vi "ReadRCMFileToTree.vi"(7 "tree control":refnum<class "TreeControl.lvclass">, 8 "error in (no error)":errorcluster) -> (0 "error out":errorcluster, 3 "rcm file path out":path)   [LabVIEW 2009]
uses:
  Support/Tree Control/Library/TreeControl.lvclass
  Support/MSXML/Public/MSXML Document/msxml document.lvclass
  Support/MSXML/Public/MSXML Node/msxml node.lvclass
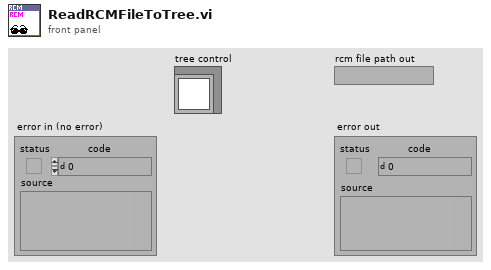
[diagram p1: front panel]
types:
  T1 = typedef "MSXML.lvlib/Attributes__slk_msxml.ctl" = T2[]
  T2 = typedef "MSXML.lvlib/Attribute__slk_msxml.ctl" = cluster{"name":string, "value":string}
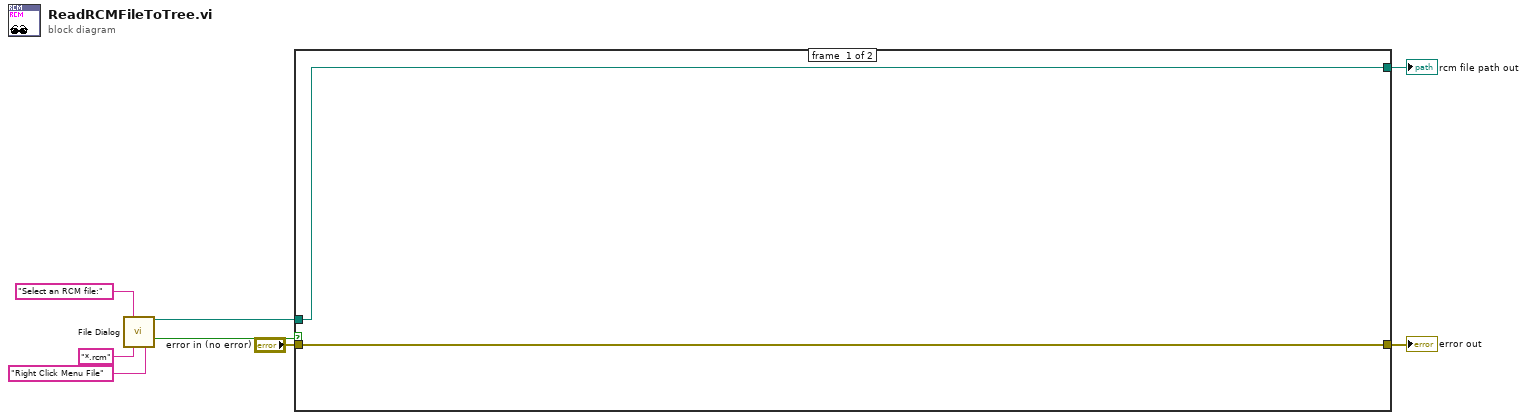
[diagram p0: block diagram]
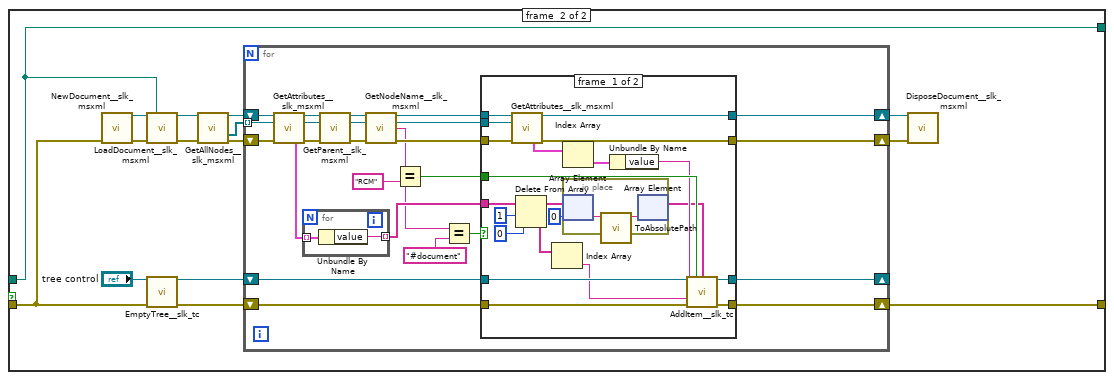
[diagram p2: hidden frame]
diagram:
  n1 = call "File Dialog"("prompt"="Select an RCM file:", "pattern (all files)"="*.rcm", "pattern label"="Right Click Menu File") -> ("selected path"=w8:path, "cancelled"=w3:bool)  [unwired: 9 in, 2 out]
  n2 = case shown="False" w3 {
    tunnel: "error in (no error)" -> [w10 w21]
    tunnel: w8 -> [w9 w23]
    tunnel: [w10 w11] -> w1
    tunnel: [w9 w23] -> w2
    frame #0 {
    }
    frame #1 {
      n3 = call "NewDocument__slk_msxml.vi"("error in (no error)"=w21) -> ("document out"=w24:refnum<class "msxml document.lvclass">, "error out"=w25:errorcluster)  [unwired: 13 in]
      n4 = call "LoadDocument__slk_msxml.vi"("document in"=w24, "xml document path in"=w23, "error in (no error)"=w25) -> ("document out"=w20:refnum<class "msxml document.lvclass">, "error out"=w19:errorcluster)  [unwired: 11 in]
      n5 = call "EmptyTree__slk_tc.vi"("tree control in"="tree control", "error in (no error)"=w21) -> ("tree control out"=w16:refnum<class "TreeControl.lvclass">, "error out"=w15:errorcluster)  [unwired: 11 in, 1 out]
      n6 = call "GetAllNodes__slk_msxml.vi"("document in"=w20, "error in (no error)"=w19) -> ("document out"=w18:refnum<class "msxml document.lvclass">, "nodes output"=w14:refnum<class "msxml node.lvclass">[], "error out"=w17:errorcluster)  [unwired: 10 in, 1 out]
      n7 = for {
        shift-right: [w30] -> w13
        shift-left: w18 -> [w50]
        shift-right: [w29] -> w12
        shift-left: w17 -> [w49]
        shift-right: [w32] -> _
        shift-left: w16 -> [w46]
        shift-right: [w31] -> w11
        shift-left: w15 -> [w45]
        tunnel: w14 -> [w48] mode=indexing
        n8 = call "GetAttributes__slk_msxml.vi"("document in"=w50, "node in"=w48, "error in (no error)"=w49) -> ("document out"=w44:refnum<class "msxml document.lvclass">, "node out"=w42:refnum<class "msxml node.lvclass">, "attributes"=w47:T1, "error out"=w43:errorcluster)  [unwired: 9 in]
        n9 = for {
          tunnel: w47 -> [w79] mode=indexing
          tunnel: [w78] -> w33 mode=indexing
          n10 = Unbundle By Name(w79) -> ("value"=w78:string)
        }
        n11 = call "GetParent__slk_msxml.vi"("document in"=w44, "child node in"=w42, "error in (no error)"=w43) -> ("document out"=w41:refnum<class "msxml document.lvclass">, "parent node out"=w40:refnum<class "msxml node.lvclass">, "error out"=w39:errorcluster)  [unwired: 10 in]
        n12 = call "GetNodeName__slk_msxml.vi"("document in"=w41, "node in"=w40, "error in (no error)"=w39) -> ("document out"=w36:refnum<class "msxml document.lvclass">, "node out"=w34:refnum<class "msxml node.lvclass">, "node name"=w27:string, "error out"=w35:errorcluster)  [unwired: 9 in]
        n13 = Equal?(x=w27, y="RCM") -> (x = y?=w37:bool)
        n14 = Equal?(x=w27, y="#document") -> (x = y?=w28:bool)
        n15 = case shown="False" w28 {
          tunnel: w46 -> [w71 w75]
          tunnel: w45 -> [w70 w74]
          tunnel: w37 -> [w69 _]
          tunnel: w36 -> [w68 w77]
          tunnel: w35 -> [w67 w76]
          tunnel: w34 -> [w66 _]
          tunnel: w33 -> [w62 _]
          tunnel: [w59 w75] -> w32
          tunnel: [w58 w74] -> w31
          tunnel: [w57 w77] -> w30
          tunnel: [w56 w76] -> w29
          frame #0 {
            n16 = call "GetAttributes__slk_msxml.vi"("document in"=w68, "node in"=w66, "error in (no error)"=w67) -> ("document out"=w57:refnum<class "msxml document.lvclass">, "attributes"=w65:T1, "error out"=w56:errorcluster)  [unwired: 9 in, 1 out]
            n17 = Delete From Array(array=w62, length=1, index=0) -> (deleted portion=w55:string[], array with subset deleted=w53:string[])
            n18 = Index Array(array=w55) -> (element=w54:string)  [unwired: 1 in]
            n19 = Index Array(array=w65) -> (element=w64:T2)  [unwired: 1 in]
            n20 = in-place {
              n21 = in-place-array #1(w53, 0) -> (w73:string)
              n22 = call "ToAbsolutePath.vi"("relative path"=w73) -> ("absolute path"=w72:string)  [unwired: 10 in]
              n23 = in-place-array #1(w72) -> (w52:string[])  [unwired: 1 out]
            }
            n24 = Unbundle By Name(w64) -> ("value"=w63:string)
            n25 = call "AddItem__slk_tc.vi"("tree control in"=w71, "make top level? (F)"=w69, "parent tag (current tag)"=w63, "new text"=w54, "error in (no error)"=w70, "column text {#1 and greater} (empty)"=w52) -> ("tree control out"=w59:refnum<class "TreeControl.lvclass">, "error out"=w58:errorcluster)  [unwired: 7 in, 1 out]
          }
          frame #1 {
          }
        }
      }
      n26 = call "DisposeDocument__slk_msxml.vi"("document in"=w13, "error in (no error)"=w12) -> ()  [unwired: 13 in, 1 out]
    }
  }
  "error out" <- w1
  "rcm file path out" <- w2
